vi "UpdateLaser.vi"(0 "Experiment in":refnum<class "Experiment.lvclass">, 5 "WV":dbl, 7 "GDD":dbl, 9 "Possition":dbl, 11 "error in (no error)":errorcluster) -> (4 "Experiment out":refnum<class "Experiment.lvclass">, 15 "error out":errorcluster)   [LabVIEW 2014, in "Experiment.lvclass"]
uses:
  Experiment.lvclass
  Experiment.lvclass/Experiment.ctl
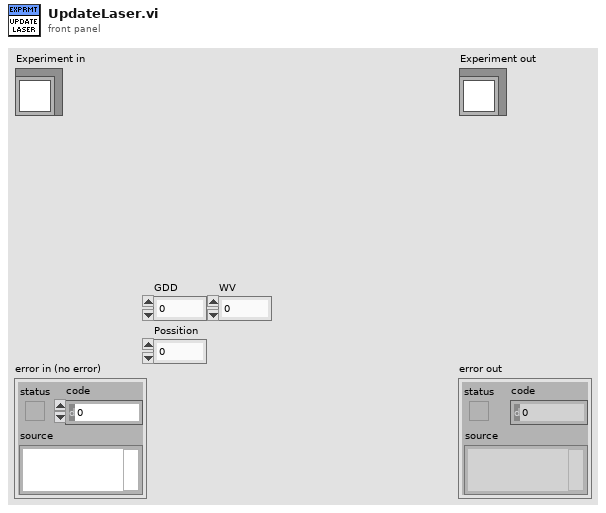
[diagram p1: front panel]
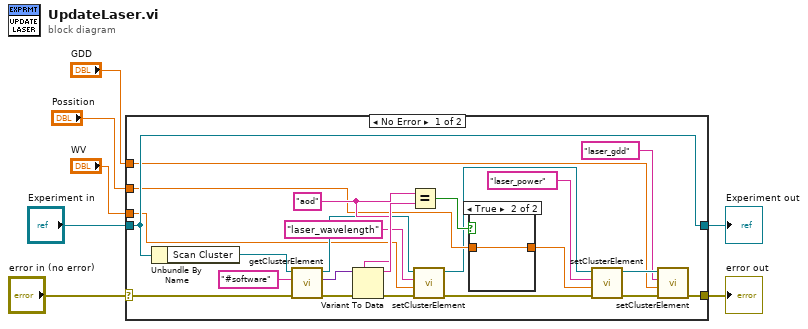
[diagram p0: block diagram]
diagram:
  n1 = case shown="No Error" "error in (no error)" {
    selector: "error in (no error)" -> [w23 w33]
    tunnel: [w14 w33] -> w6
    tunnel: [w30 w32] -> w4
    tunnel: "Experiment in" -> [w30 w32]
    tunnel: "Possition" -> [w22 _]
    tunnel: "GDD" -> [w8 _]
    tunnel: "WV" -> [w10 _]
    frame No Error {
      w26 = "aod"
      n2 = Unbundle By Name(w30) -> ("Scan Cluster"=w24:refnum<vi>)
      n3 = call "getClusterElement.vi"("error in (no error)"=w23, "Label.Text"="#software", "reference"=w24) -> ("error out"=w21:errorcluster, "Value"=w28:variant, "reference 2"=w20:refnum<vi>)  [unwired: 6 in]
      n4 = Variant To Data(error in=w21, type=w26, Variant=w28) -> (data=w27:string, error out=w15:errorcluster)
      n5 = Equal?(x=w26, y=w27) -> (x = y?=w25:bool)
      n6 = call "setClusterElement.vi"("error in (no error)"=w15, "Value"=w10, "Label.Text"="laser_wavelength", "reference"=w20) -> ("error out"=w16:errorcluster, "reference 2"=w19:refnum<vi>)  [unwired: 6 in]
      n7 = case shown="True" w25 {
        tunnel: w22 -> [_ w31]
        tunnel: [_ w31] -> w9
        frame False {
        }
        frame True {
        }
      }
      n8 = call "setClusterElement.vi"("error in (no error)"=w16, "Value"=w9, "Label.Text"="laser_power", "reference"=w19) -> ("error out"=w17:errorcluster, "reference 2"=w18:refnum<vi>)  [unwired: 6 in]
      n9 = call "setClusterElement.vi"("error in (no error)"=w17, "Value"=w8, "Label.Text"="laser_gdd", "reference"=w18) -> ("error out"=w14:errorcluster)  [unwired: 6 in, 1 out]
    }
    frame Error {
    }
  }
  "error out" <- w6
  "Experiment out" <- w4
